vi "Write ref.vi"(8 "error in (no error)":errorcluster, 10 "ref":refnum<k24>, 11 "DapperRow in":refnum<class "DapperRow.lvclass">) -> (0 "error out":errorcluster, 3 "DapperRow out":refnum<class "DapperRow.lvclass">)   [LabVIEW 2020, in "ORM_Dapper.lvlib" / "DapperRow.lvclass"]
uses:
  DapperRow.lvclass
  DapperRow.lvclass/DapperRow.ctl
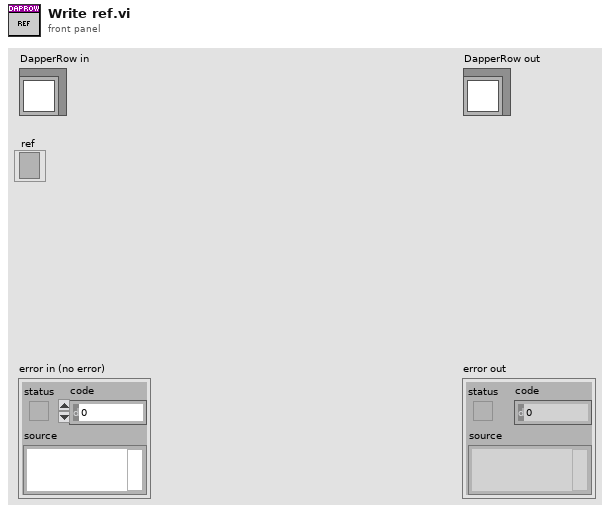
[diagram p1: front panel]
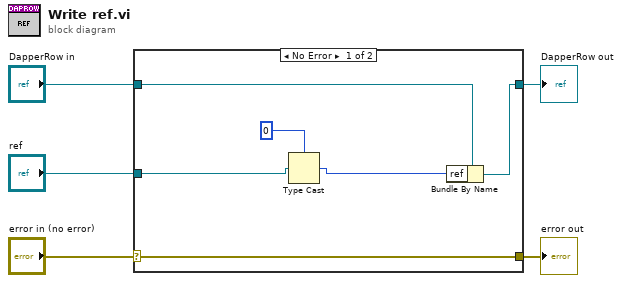
[diagram p0: block diagram]
diagram:
  n1 = case shown="No Error" "error in (no error)" {
    selector: "error in (no error)" -> [w11 w12]
    tunnel: [w11 w12] -> w4
    tunnel: [w9 w13] -> w2
    tunnel: "DapperRow in" -> [w10 w13]
    tunnel: "ref" -> [w8 _]
    frame No Error {
      n2 = Type Cast(type=u64 0 ("ref"), x=w8) -> (*(type *) &x=w6:u64)
      n3 = Bundle By Name(cluster=w10, "ref"=w6) -> (w9:refnum<class "DapperRow.lvclass">)
    }
    frame Error {
    }
  }
  "error out" <- w4
  "DapperRow out" <- w2
